vi "Example showing how single values are equivelent to 1-element arrays.vi"() -> ()   [LabVIEW 2019]
doc: "Example showing how indiviual JSON Values can be gotten as 1-element Arrays of LabVIEW types.\n\nThis suppoprts JSON that sometimes has arrays of multiple items, but also can have individual items."
uses:
  aabef2c6-47df-460d-9fc9-1e0b29759df5.vi
  vi.lib/JDP Science/JSONtext/JSON text to Variant.vi
  vi.lib/JDP Science/JSONtext/LVClass Serializer/JSONtext LVClass Serializer.lvclass
panel:
  in  "JSON in":string[](array[string])=["{\n\"Number\":123\n\"Text\":\"abc\"\n\"Obj\":{\"a\":1}\n}", "{\n\"Number\":[123,456]\n\"Text\":[\"abc\",\"def\"]\n\"Obj\":[{\"a\":1},{\"b\":2}]\n}"]
  out "error out":errorcluster
  out "Data out":T1(array[cluster])
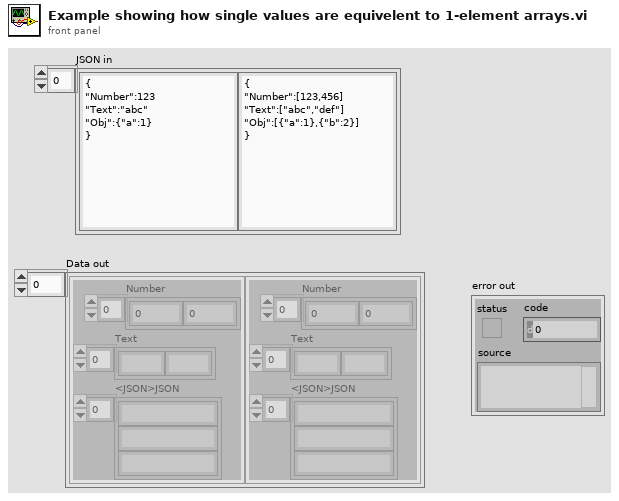
[diagram p1: front panel]
types:
  T1 = cluster{"Number":i32[], "Text":string[], "<JSON>JSON":string[]}[]
  T2 = cluster{"Number":i32[], "Text":string[], "Obj":string[]}
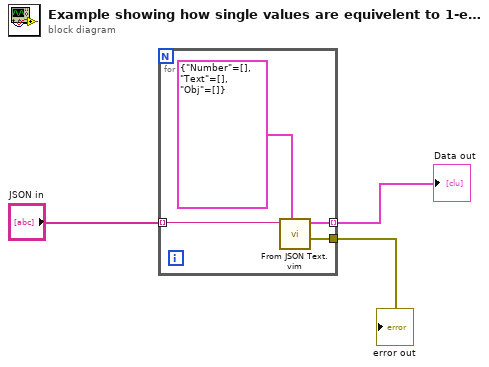
[diagram p0: block diagram]
diagram:
  n1 = for {
    tunnel: "JSON in" -> [w7] mode=indexing
    tunnel: [w6] -> w2 mode=indexing
    tunnel: [w5] -> w1
    n2 = call "From JSON Text.vim"("Data Type and Default Value"=T2 {"Number"=[], "Text"=[], "Obj"=[]}, "JSON"=w7) -> ("error out"=w5:errorcluster, "Data out"=w6:T2)  [unwired: 8 in]
  }
  "Data out" <- w2
  "error out" <- w1
